vi "SetSampleRate.vi"(8 "错误输入（无错误）":errorcluster, 10 "SampleRate":u32=100000, 11 "DevIndex":i32) -> (0 "错误输出":errorcluster, 3 "DevIndex Output":i32)   [LabVIEW 2018]
panel:
  out "ErroCode":i32
  # "SamplaRate: points/s all channels"
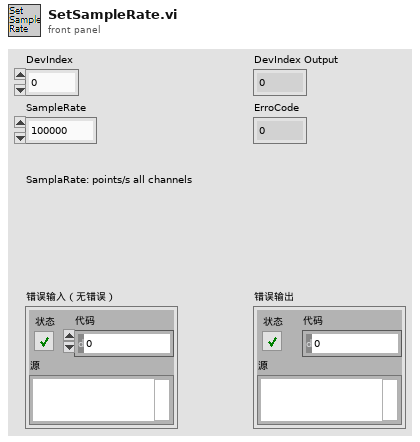
[diagram p1: front panel]
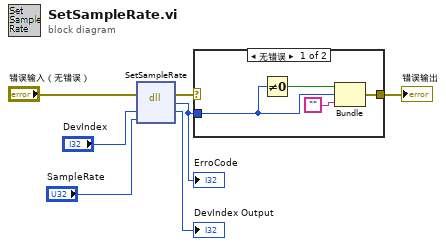
[diagram p0: block diagram]
diagram:
  n1 = dll-call lib="PTH2@abs H科研项目仅一项目程序32位usb-1000.dll" fn="SetSampleRate"(error in="错误输入（无错误）", "DevIndex"="DevIndex", "SampleRate"="SampleRate") -> (error out=w3:errorcluster, "ErroCode"=w1:i32, "DevIndex"=→"DevIndex Output":i32)  [unwired: 3 in, 1 out]
  "ErroCode" <- w1
  n2 = case shown="无错误" w3 {
    selector: w3 -> [_ w12]
    tunnel: [w9 w12] -> w2
    tunnel: w1 -> [w10 _]
    frame No Error {
      n3 = Not Equal To 0?(x=w10) -> (x != 0?=w11:bool)
      n4 = Bundle(w11, "ErroCode"=w10, "") -> (w9:cluster{bool, "ErroCode":i32, string})  [unwired: 1 in]
    }
    frame Error {
    }
  }
  "错误输出" <- w2
